vi "hse-configuration_ReadIntegerKey.vi"(8 "error in (no error)":errorcluster, 9 "Key":string, 10 "Section":string, 11 "hse-configuration in":refnum<class "hse-configuration.lvclass">) -> (0 "error out":errorcluster, 2 "Value":i32, 3 "hse-configuration out":refnum<class "hse-configuration.lvclass">)   [LabVIEW 2022 SP3, in "hse-configuration.lvclass"]
doc: "Reads the numeric configuration value (I32) identified by <b>section</b> and <b>key</b> from the configuration object\n\n____\nHAMPEL SOFTWARE ENGINEERING v3.8.0 (2023-12-18 14:41)"
uses:
  hse-configuration.lvclass
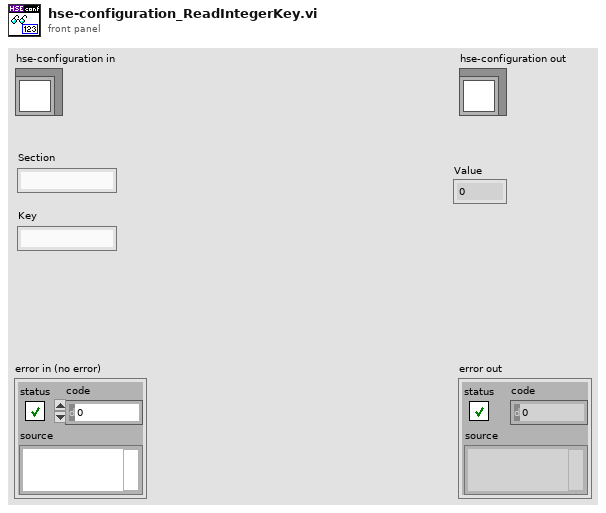
[diagram p1: front panel]
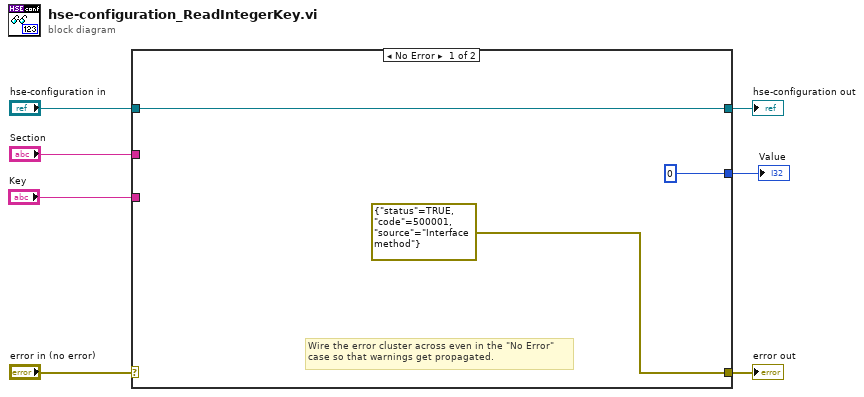
[diagram p0: block diagram]
diagram:
  n1 = case shown="No Error" "error in (no error)" {
    selector: "error in (no error)" -> [_ w12]
    tunnel: [errorcluster {"status"=TRUE, "code"=500001, "source"="Interface method"} ("error IO") w12] -> w6
    tunnel: [w10 w11] -> w4
    tunnel: "hse-configuration in" -> [w10 w11]
    tunnel: "Section" -> [_ _]
    tunnel: "Key" -> [_ _]
    tunnel: [0 _] -> w1
    frame No Error {
      # "Wire the error cluster across even in the \"No Error\"\ncase so that warnings get propagated."
    }
    frame Error {
    }
  }
  "error out" <- w6
  "hse-configuration out" <- w4
  "Value" <- w1
